vi "MenuActivation Response.vi"(8 "error in (no error)":errorcluster, 9 "Coords":T1, 10 "Menu Refnum":refnum<k9>, 11 "Editor Handler in":refnum<class "Image Editor Handler.lvclass">) -> (0 "error out":errorcluster, 3 "Editor Handler out":refnum<class "Image Editor Handler.lvclass">)   [LabVIEW 2015, in "LV Image Editor Framework.lvlib" / "Image Editor Handler.lvclass"]
uses:
  Image Editor Handler.lvclass
  <vilib>/Utility/miscctls.llb/LVPoint32TypeDef.ctl
  Image Editor Handler.lvclass/Image Editor Handler.ctl
  Forms/Shape/Shape.lvclass
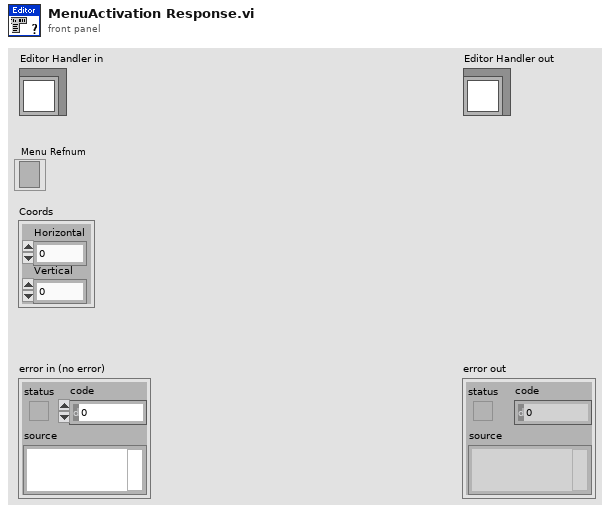
[diagram p1: front panel]
types:
  T1 = typedef "LVPoint32TypeDef.ctl" = cluster{"Horizontal":i32, "Vertical":i32}
  T2 = typedef "LVPositionTypeDef.ctl" = cluster{"Left":i32, "Top":i32}
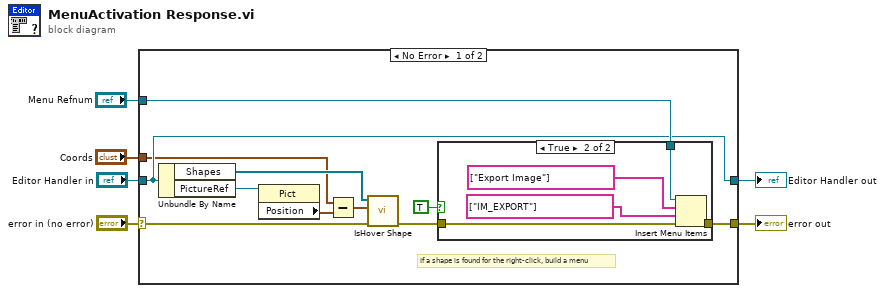
[diagram p0: block diagram]
diagram:
  n1 = case shown="No Error" "error in (no error)" {
    selector: "error in (no error)" -> [w13 w25]
    tunnel: [w16 w25] -> w5
    tunnel: [w14 w24] -> w3
    tunnel: "Editor Handler in" -> [w14 w24]
    tunnel: "Menu Refnum" -> [w17 _]
    tunnel: "Coords" -> [w10 _]
    frame No Error {
      # "If a shape is found for the right-click, build a menu"
      n2 = Unbundle By Name(w14) -> ("Shapes"=w15:refnum<data-value>[], "PictureRef"=w11:refnum<vi>)
      n3 = property class="Pict"(reference=w11) -> ("Position"=w9:T2)  [unwired: 1 in, 2 out]
      n4 = Subtract(x=w10, y=w9) -> (x-y=w8:T1)
      n5 = call "IsHover Shape.vi"("error in (no error)"=w13, "Coords"=w8, "Shape in"=w15) -> ("error out"=w12:errorcluster)  [unwired: 3 in, 5 out]
      n6 = case shown="True" TRUE {
        tunnel: w17 -> [_ w23]
        tunnel: [w18 w22] -> w16
        tunnel: w12 -> [w18 w20]
        frame False {
        }
        frame True {
          n7 = Insert Menu Items(6:w20, 7:string[] ["IM_EXPORT"] ("Tags"), 8:string[] ["Export Image"] ("Tags"), 9:w23) -> (0:w22:errorcluster)  [unwired: 2 in, 2 out]
        }
      }
    }
    frame Error {
    }
  }
  "error out" <- w5
  "Editor Handler out" <- w3
